vi "AlliGator Fit Decay.vi"(0 "Selected Plot Info + Flag":T13={"Multiplot XY Graph"=refnum, "Mouse Coordinates"={"Horizontal"=0, "Vertical"=0}, "Plot Index"=-1, "Flag"=FALSE}, 1 "Decay Fit Options & Parameters":T2 {"Fit Options"."Offset Resolution" min=0.0; "Fit Options"."Period" min=0.0; "Fit Options"."Min Decay Percentile" min=0.0 max=1.0; "Fit Options"."Max Decay Percentile" min=0.0 max=100.0; "Fit Parameter Constraints"."Max Value" format="%#.3g"; "Fit Parameter Constraints"."Min Value" format="%#.3g"}, 5 "Current Decay Name":string, 7 "Current Decay":T16, 9 "Reference Decay":T16, 11 "error in (no error)":errorcluster, 12 "Use Legacy Fitting Approach":bool) -> (2 "Decay Fit Options & Parameters (out)":T2 {"Fit Options"."Offset Resolution" min=0.0; "Fit Options"."Period" min=0.0; "Fit Options"."Min Decay Percentile" min=0.0 max=1.0; "Fit Options"."Max Decay Percentile" min=0.0 max=100.0; "Fit Parameter Constraints"."Max Value" format="%#.3g"; "Fit Parameter Constraints"."Min Value" format="%#.3g"}, 3 "Output Plots":T1(array[cluster]), 4 "Best Fit Parameters (All)":dbl[](array[numeric]), 6 "Delta Best Fit Parameters (All)":dbl[](array[numeric]), 8 "R^2":dbl, 10 "Reduced Chi^2":dbl, 13 "Output Plot Names":string[](array[string]), 14 "Fit Output Message":string, 15 "Error Out":errorcluster)   [LabVIEW 2021, in "AlliGator Decay Analysis.lvlib" / "AlliGator Decay Fit.lvlib"]
doc: "VI implementing single decay fit with either a single or double exponential model with IRF convolution (or in the absence of IRF, without convolution)."
uses:
  AlliGator Decay Fit.lvlib
  <vilib>/Analysis/Matrix/Datatypes/RealMatrix.ctl
  Graphs/XY Graph/XY Graph Selected Plot Info+Flag.ctl
  Graphs/XY Graph/XY Graph Refnum.ctl
  <vilib>/Utility/miscctls.llb/LVPoint32TypeDef.ctl
  AlliGator Decay Fit Options & Parameters v2.ctl
  Fits/IRF(X)PSED/Decay Fit Options v2.ctl
  Fits/Decay Convolution/Decay Model.ctl
  Fits/Residual Type.ctl
  Fits/IRF(X)PSED/Fit Weights Type.ctl
  Fits/Non-linear Fitting Method v2.ctl
  Fits/Fit Calculation Method.ctl
  Fits/Non-linear Fitting Algorithm.ctl
  AlliGator Decay Fit Parameter Constraints 2.ctl
  Fits/IRF(X)PSED/Decay Fit Parameters In List.ctl
  Fits/IRF(X)PSED/MLE Baseline Offset Type.ctl
  AlliGator Settings List.ctl
  AlliGator Variables List.ctl
  Fits/IRF(X)PSED/MLE Fit Options.ctl
  Graphs/Get Plot at Mouse Click (XY Graph)/Get Plot at Mouse Click [AAC].vi
  <vilib>/Utility/error.llb/Error Cluster From Error Code.vi
  Fits/Decay Convolution/LM model function and gradient (1-Exp, Convolved, Periodic, Fixed Parameters) v3.vi
  Fits/Decay Convolution/LM model function and gradient (2-Exp, Convolved, Periodic, Fixed Parameters) v3.vi
  Fits/Abort Fit Global.vi
  Graphs/XY Graph/XY Graph Add Multiplots with Names.vi
  <vilib>/ErrorRing/Error Ring.xnode
  Graphs/Graphs.lvlib
  Graphs/XY Graph/XY Graph Add-Ons.lvlib
  AlliGator Settings.lvlib
  Fits/Fits.lvlib
  AlliGator Globals, Variables & Constants.lvlib
  Time/Time.lvlib
  Strings/Strings.lvlib
  <vilib>/Analysis/Matrix/NI_Matrix.lvlib
  AlliGator Decay Fit Parameter Map.lvlib
panel:
  in  "Reset Fit Options & Parameters":bool
  out "Covariance":T17
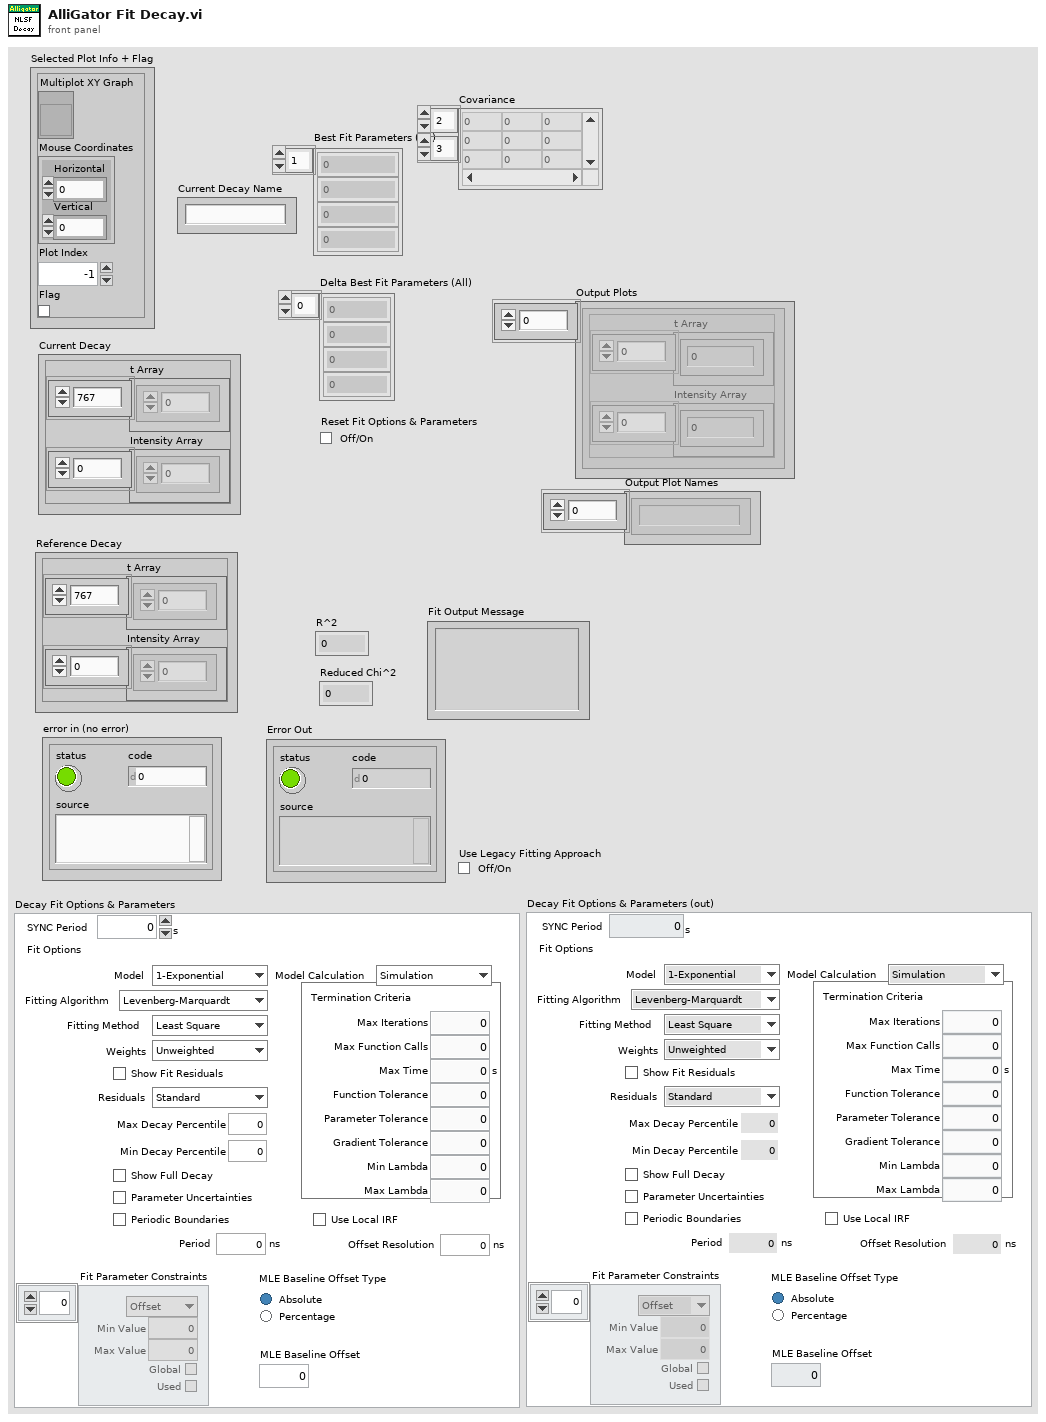
[diagram p1: front panel]
types:
  T1 = cluster{"t Array":dbl[], "Intensity Array":dbl[]}[]
  T2 = typedef "AlliGator Decay Fit Parameter Map.lvlib/AlliGator Decay Fit Options & Parameters v2.ctl" = cluster{"SYNC Period":dbl[unit], "Fit Options":T3, "Fit Parameter Constraints":T10[], "MLE Baseline Offset":dbl, "MLE Baseline Offset Type":T12}
  T3 = typedef "Fits.lvlib/Decay Fit Options v2.ctl" = cluster{"Show Fit Residuals":bool, "Fit Model":T4, "Residual Type":T5, "Max Decay Percentile":dbl, "Min Decay Percentile":dbl, "Show Full Decay":bool, "Weights":T6, "Fitting Method":T7, "Compute Parameter Uncertainties":bool, "Periodic Boundaries":bool, "Model Calculation":T8, "Period":dbl[unit], "Termination Criteria":cluster{"Max Iterations":i32, "Max Function Calls":i32, "Max Time":dbl[unit], "Function Tolerance":dbl, "Parameter Tolerance":dbl, "Gradient Tolerance":dbl, "Min Lambda":dbl, "Max Lambda":dbl, "Initial Tick Count":u32}, "Offset Resolution":dbl[unit], "Use Local IRF":bool, "Fitting Algorithm":T9}
  T4 = typedef "Fits.lvlib/Decay Model.ctl" = enum16{"1-Exponential", "2-Exponentials"}
  T5 = typedef "Fits.lvlib/Residual Type.ctl" = enum16{"Standard", "Normalized", "Reduced"}
  T6 = typedef "Fits.lvlib/Fit Weights Type.ctl" = enum16{"Unweighted", "1/Variance", "Best of All"}
  T7 = typedef "Fits.lvlib/Non-linear Fitting Method v2.ctl" = enum16{"Least Square", "Least Absolute Residual", "Bisquare", "MLE", "-", "Best of All"}
  T8 = typedef "Fits.lvlib/Fit Calculation Method.ctl" = enum16{"Simulation", "Convolution", "Integration"}
  T9 = typedef "Fits.lvlib/Non-linear Fitting Algorithm.ctl" = enum16{"Levenberg-Marquardt", "Trust-Region Dogleg"}
  T10 = typedef "AlliGator Decay Analysis.lvlib/AlliGator Decay Fit.lvlib/AlliGator Decay Fit Parameter Constraints 2.ctl" = cluster{"Fit Parameter":T11, "Min Value":dbl, "Max Value":dbl, "Global":bool, "Used":bool}
  T11 = typedef "Fits.lvlib/Decay Fit Parameters In List.ctl" = enum16{"Offset", "Baseline", "A_1", "tau_1", "A_2", "tau_2"}
  T12 = typedef "Fits.lvlib/MLE Baseline Offset Type.ctl" = enum32{"Absolute", "Percentage"}
  T13 = typedef "XY Graph Add-Ons.lvlib/XY Graph Selected Plot Info+Flag.ctl" = cluster{"Multiplot XY Graph":T14, "Mouse Coordinates":T15, "Plot Index":i32, "Flag":bool}
  T14 = typedef "XY Graph Add-Ons.lvlib/XY Graph Refnum.ctl" = refnum<vi>
  T15 = typedef "LVPoint32TypeDef.ctl" = cluster{"Horizontal":i32, "Vertical":i32}
  T16 = cluster{"t Array":dbl[], "Intensity Array":dbl[]}
  T17 = typedef "NI_Matrix.lvlib/RealMatrix.ctl" = dbl[][]
  T18 = typedef "AlliGator Settings.lvlib/AlliGator Settings List.ctl" = enum16{"GUI:Visible Settings Tab", "GUI:Last Run Version", "Source Image:Use Image Histogram for Contrast", "Source Image:Low Count Pixels Rejection Options", "Source Image:High Count Pixels Rejection Options", "Source Image:Use Image Brightness", "Source Image:Blend Overlay with Image Background", "Source Image:Use Fixed ROI Diameter", "Source Image:ROI Diameter", "Source Image:ROI Center Color", "Source Image:Peak Threshold", "Source Image:Intensity Threshold", "Source Image:Image Binning Options", "Source Image:Image Smoothing Options", "Source Image:Image Histogram Active", "Source Image:Invert Binary Mask", "Source Image:Hot Pixel Removal", "Source Image:Overlay Analyzed ROI Center", "Source Image:Auto-Adjust Contrast", "Source Image:Histogram Lower Percentile", "Source Image:Histogram Upper Percentile", "Source Image:Save Source Image", "Source Image:Scale Bar Options", "Source Image:Image Resolution (Pixel Size)", "Source Image:Flatfield Correction", "Source Image:Show Dead Left Columns Correction", "Source Image:Dead Left Columns Correction", "Source Image:Image Pre-Processing Operations Order", "Data Information:Gate Width", "Data Information:Nanotime Gate Separation", "Data Information:Macrotime Gate Separation", "Data Information:Gate Step", "Data Information:# Gates", "Data Information:Gate Image Exposure", "Data Information:Gate Image Integration", "Data Information:Gates to Skip", "Data Information:Gates to Keep", "Data Information:Define Gates to", "Data Information:Channel Name", "Data Information:Available Channel Names", "Data Information:Channel Arithmetic", "Data Information:Background File Subtraction", "Data Information:Background File", "Data Information:Background Scaling Factor", "Data Information:Background Pile-up Correction", "Data Information:Background Pixel Well Capacity", "Data Information:Laser Period", "Data Information:SYNC Period", "Data Information:Pile-up Correction", "Data Information:Pixel Well Capacity", "Data Information:Dataset Scaling Factor", "Fluorescence Decay_Decay Pre-Processing:Reverse Gates", "Fluorescence Decay_Decay Pre-Processing:Verbose Decay Pre-Processing", "Fluorescence Decay_Decay Pre-Processing:Use Decay Pre-Processing", "Fluorescence Decay_Decay Pre-Processing:Background Subtraction", "Fluorescence Decay_Decay Pre-Processing:Background Definition Range", "Fluorescence Decay_Decay Pre-Processing:Baseline Subtraction Method", "Fluorescence Decay_Decay Pre-Processing:Decay Pre-Processing Operations Order", "Fluorescence Decay_Decay Pre-Processing:Smoothing Parameter", "Fluorescence Decay_Decay Pre-Processing:Shift Decay", "Fluorescence Decay_Decay Pre-Processing:Decay Shift Parameters", "Fluorescence Decay_Decay Pre-Processing:Fold Decay", "Fluorescence Decay_Decay Pre-Processing:# Folds", "Fluorescence Decay_Decay Pre-Processing:1-Normalize Decay", "Fluorescence Decay_Decay Pre-Processing:[0-1]-Normalize Decay", "Fluorescence Decay_Decay Pre-Processing:Smoothen Decay", "Fluorescence Decay_Decay Pre-Processing:Extrapolate Decay", "Fluorescence Decay_Decay Pre-Processing:Use Periodicity", "Fluorescence Decay_Decay Pre-Processing:Use Cursors", "Fluorescence Decay_Decay Pre-Processing:Tail Fraction", "Fluorescence Decay_Decay Pre-Processing:Head Fraction", "Fluorescence Decay_Decay Pre-Processing:Additional Points", "Fluorescence Decay_Decay Pre-Processing:Straighten Decay", "Fluorescence Decay_Decay Pre-Processing:Constant Background", "Fluorescence Decay_Decay Pre-Processing:Pixel-Normalize Decay", "Fluorescence Decay_Advanced Analysis:Extract IRF instead of Decay", "Fluorescence Decay_Advanced Analysis:IRF Extraction Options", "Fluorescence Decay_Advanced Analysis:IRF Optimization Options", "Fluorescence Decay_Advanced Analysis:Square Pulse Options", "Fluorescence Decay_Advanced Analysis:IRF Order", "Fluorescence Decay_Advanced Analysis:IRF Time Constants", "Fluorescence Decay_Advanced Analysis:Wavelet Analysis Options", "Fluorescence Decay_Advanced Analysis:Average Lifetime Options", "Fluorescence Decay_Fit Options:Fit Options", "Fluorescence Decay_Fit Options:Use Legacy Fitting Approach", "Fluorescence Decay_Fit Options:Use Data Information Laser Period", "Fluorescence Decay_Fit Parameters:Displayed Fit Parameters", "Fluorescence Decay_Fit Parameters:Fit Parameter Constraints", "Fluorescence Decay_Fit Parameters:Export Tabulated Results", "Fluorescence Decay_Fit Parameters:MLE Baseline Offset Type", "Fluorescence Decay_Fit Parameters:MLE Baseline Offset", "Fluorescence Decay_Fit Parameters:Guess Parameter Names", "Fluorescence Decay_Fit Parameters:Guess Parameter Values", "Fluorescence Decay_Fit Parameters:Guess Parameters Options", "Fluorescence Decay_Styles:Show Last Decay Only", "Fluorescence Decay_Styles:Decay Graph Color Array", "Fluorescence Decay:Decay Graph Active", "Fluorescence Decay Statistics:Min Peak Value", "Fluorescence Decay Statistics:Reject Low Decay Peak Pixels", "Fluorescence Decay Statistics:Reject High Decay Peak Pixels", "Fluorescence Decay Statistics:Max Peak Value", "Time Traces:Use File Timestamp", "Time Traces:Time Step", "Time Traces:Use Intensity Correction File", "Time Traces:Intensity Correction File", "Phasor Plot:Phasor Plot Smoothing Options", "Phasor Plot:Phasor Plot Size", "Phasor Plot:Phasor Plot Graphics Options", "Phasor Plot:Cumulative Phasor Plot", "Phasor Plot:Use Phasor Brightness", "Phasor Plot:Blend Overlay with Phasor Background", "Phasor Plot:Save Phasor Plot", "Phasor Plot:Show References", "Phasor Plot:Phasor Ratio Decay Range", "Phasor Plot:Exponential Fading", "Phasor Plot:Phasor Ratio Reference Colors", "Phasor Plot:Reference Radius", "Phasor Plot:Show Color Map Vertices", "Phasor Plot:Phasor Plot Active", "Phasor Plot:Phasor Ratio Color Map Type", "Phasor Plot:Phasor Ratio Color Map", "Phasor Plot:Phasor Ratio Display Range", "Phasor Plot:Selected Image ROI(s)", "Phasor Plot:All Image ROIs", "Phasor Plot:Selected Phasor Plot ROI(s)", "Phasor Plot:All Phasor Plot ROIs", "Phasor Plot:Phasor Ratio Color-Coded Quantity", "Phasor Plot:Store Phasor Harmonics", "Phasor Plot:Draw Reference Segment", "Phasor Plot:User-Defined Quantity", "Phasor Graph:Phasor Frequency", "Phasor Graph:Phasor Ratio Type", "Phasor Graph:Pixel-level Phasor Computation", "Phasor Graph:Save Phasor Graph", "Phasor Graph:Phasor Graph Active", "Phasor Graph:Phasor SDV Options", "Phasor Calibration:Use Backup Calibration if needed", "Phasor Graph:Define Shortest Lifetime as", "Phasor Calibration:Backup Calibration Type", "Phasor Calibration:Calibration Type", "Phasor Calibration:Calibration Lifetime", "Phasor Calibration:Calibration Map Algorithm", "Single-Exponential Phasor Locus (SEPL):Gate Parameters", "Single-Exponential Phasor Locus (SEPL):User-defined Gate", "Single-Exponential Phasor Locus (SEPL):User-defined IRF", "Single-Exponential Phasor Locus (SEPL):Phasor Parameters", "Single-Exponential Phasor Locus (SEPL):Decay & IRF Parameters", "Single-Exponential Phasor Locus (SEPL):Display Parameters", "Lifetime Analysis:Decay Analysis Parameters", "Lifetime Analysis:Lifetime Map Active", "Plugins:Python Settings", "Miscellaneous:Verbose Mode", "Miscellaneous:Beep after Script", "Miscellaneous:Saved Image File Format", "Miscellaneous:Exported Gate Image Settings", "Miscellaneous:Include Loading in Timing", "Miscellaneous:Verbose Settings Mode", "Miscellaneous:Histogram Options", "Miscellaneous:Beep on Error", "Miscellaneous:# Logical Processors Used", "Miscellaneous:ROI Description Max Characters", "Miscellaneous:Verbose Error Mode", "Miscellaneous:Transparent Mask Color"}
  T19 = cluster{"X Array out":dbl[], "Y Array out":dbl[]}
  T20 = typedef "AlliGator Globals, Variables & Constants.lvlib/AlliGator Variables List.ctl" = enum16{"---- GUI ----", "Initialization Status", "State Indicators Refnum", "Original AlliGator Menu Items", "Current Action Loop State", "Script in progress", "Playback", "Loop Playback", "Search ROI Used", "Search ROI", "Decay Graph Max Legend Size", "Intensity Graph Max Legend Size", "Decay Statistics Graph Max Legend Size", "Phasor Graph Max Legend Size", "Phasor Ratio Graph Max Legend Size", "Lifetime Graph Max Legend Size", "---- Files ----", "Export Dataset Frames as Individual Files", "Show Batch Export Help Balloons", "Frames in Dataset", "ptu File Frame Start Indices", "Current Frame in Dataset", "Current Frame Timestamp", "------ Python Plugins ------", "Python Plugins Information", "Python Session", "Valid Python Session?", "---- Source Image ----", "Dataset Loaded", "Dataset Metadata", "Dataset Channel", "Dataset Data Description", "Background Dataset Metadata", "Background Dataset Channel", "Background Dataset Data Description", "Background File Subtraction", "Background File Path", "Background File Pile-up Correction", "Background File Pixel Well Capacity", "Background File Scaling Factor", "Source Image ROIs", "Current Source Image ROI", "Source Image ROI Event Refnum", "X_Source Image Display Range", "X_Source Image Palette Information", "Source Image Palette List", "Source Image Scale", "Current Dataset Load Settings", "Source Image:ROI Overlay Color", "---- Image Profile Window ----", "Image Profile:Overlay ROI in Source Image", "Image Profile Window Event Refnum", "Image Profile:IntensityType", "Image Profile:Intensity Average Type", "Image Profile:Intensity-weighted SDV", "Image Profile:Box Profile Type", "Image Profile Window Open", "Image Profile:Plotted Fit Parameter", "X_Type of Displayed Image", "X_Time Gate Slider", "Dataset Path", "Source Image Overlay to Erase", "Is Displayed Image Accumulated", "White Light Image Modified", "Mask Image Modified", "Macrotime Gate Separation", "------ Phasor Graph -------", "Phasor Graph:Show Line", "---- Phasor Plot ---", "Phasor Plot Parameters Changed", "FLI Dataset Modified since last Phasor Plot Calculation", "Phasor Harmonics Data", "Selected Phasor Harmonics", "Phasor Harmonic Manager Event Refnum", "Phasor Plot ROIs", "Current Phasor Plot ROI", "Phasor Plot ROI Event Refnum", "Phasor Plot Image Reference Points", "Phasor Plot Computed", "Phasor Plot Palette Information", "Phasor Plot Palette List", "Phasor Ratio Palette Information", "Phasor Ratio Palette List", "Phasor Image Scale", "Phasor Plot Image Overlay to Erase", "Phasor Plot Image Elements to Update", "Current Phasor Plot Calculation Parameters", "Current Phasor Calibration Options", "Reset Cumulated Phasor Plot", "Phasor Ratio Reference 1", "Phasor Ratio Lifetime Reference 1", "Phasor Ratio Reference 1 Frequency", "Phasor Ratio Reference 2", "Phasor Ratio Lifetime Reference 2", "Phasor Ratio Reference 2 Frequency", "---- Decay Analysis ----", "Number of Selected Decays to Fit", "LS Fit Results", "LAR Fit Results", "BS Fit Results", "Last Decay Max - Min", "Best Fit Parameters", "Best Fit Parameter Names", "Actual Size X", "Actual Size Y", "Binning X", "Binning Y", "Actual # Gates", "Dataset Number", "Gates to...", "Gates Skipped", "Gates to keep", "Gate Step", "Gate Separation", "Reversed Gates", "Pile-up Correction", "Pixel Well Capacity", "Background Subtracted", "Background Subtraction Method", "Background Definition Range", "Background File (deprecated)", "Number of Dataset Accumulated", "Array of Accumulated Dataset Paths", "Do Averaged Datasets", "Destination File Path", "Process Plot Target", "Use 1/D as Phasor Frequency", "---- Decay Fit Parameter Map -----", "Decay Fit Parameter Map Palette Information", "Decay Fit Parameter Map Palette List", "Local Decay Graph Window Event Refnum", "------- Local Decay Window ---------", "Use normalized IRF for convolution", "----- Miscellaneous ----", "Skippable Dialog Windows Status"}
  T21 = typedef "Fits.lvlib/MLE Fit Options.ctl" = cluster{"MLE Baseline Offset":dbl, "MLE Baseline Offset Type":T12}
  T22 = typedef "Fits.lvlib/Decay Fit Parameter Constraints Arrays.ctl" = cluster{"Parameter Bounds (Fix+Fit)":cluster{"parameter minimum":dbl[], "parameter maximum":dbl[]}, "Fitted Parameters":T11[], "Fixed Parameters":T11[], "Fit Model":T4}
  T23 = typedef "Graphs.lvlib/Plot Range.ctl" = cluster{"X Minimum":dbl, "X Maximum":dbl, "Y Minimum":dbl, "Y Maximum":dbl}
  T24 = cluster{"parameter minimum":dbl[], "parameter maximum":dbl[]}
  T25 = typedef "Fits.lvlib/Non-linear Fit Output v3.ctl" = cluster{"best nonlinear fit":dbl[], "best fit parameters":dbl[], "R^2":dbl, "RMSE":dbl, "error out":errorcluster, "Fitting Method":T26, "number of function calls":i32, "number of iterations":i32, "covariance":T17, "Chi 2":dbl, "DOF":i32, "Fit Convergence Criterion":T27, "Fitting Algorithm":T9, "Weighted Fit":bool, "Gradient":dbl, "|Delta Chi 2|":dbl, "|Delta Chi 2|/Chi 2":dbl, "Max |Delta a| /|a|":dbl, "Lambda":dbl, "RSS":dbl, "AIC":dbl, "BIC":dbl, "Max number of function calls":i32, "Max number of iterations":i32, "IRF":T28, "IRF Normalization Factor":dbl, "Decay Normalization Factor":dbl}
  T26 = typedef "Fits.lvlib/Nonlinear Fit Method.ctl" = enum16{"Least Square", "Least Absolute Residual", "Bisquare", "MLE"}
  T27 = typedef "Fits.lvlib/Convergence Criteria.ctl" = enum16{"Continue", "Tolerances Exceeded", "Max Time Exceeded", "Max Iterations Exceeded", "Max Function Evaluations Exceeded", "Scale Range Exceeded"}
  T28 = typedef "XY Graph Add-Ons.lvlib/XY Plot Data.ctl" = cluster{"X Array":dbl[], "Y Array":dbl[]}
  T29 = typedef "AlliGator Decay Analysis.lvlib/AlliGator Decay Fit.lvlib/AlliGator Guess Parameters Options.ctl" = enum16{"Numerically estimated", "User-provided", "User-provided (normalized)", "Last valid fitted parameters"}
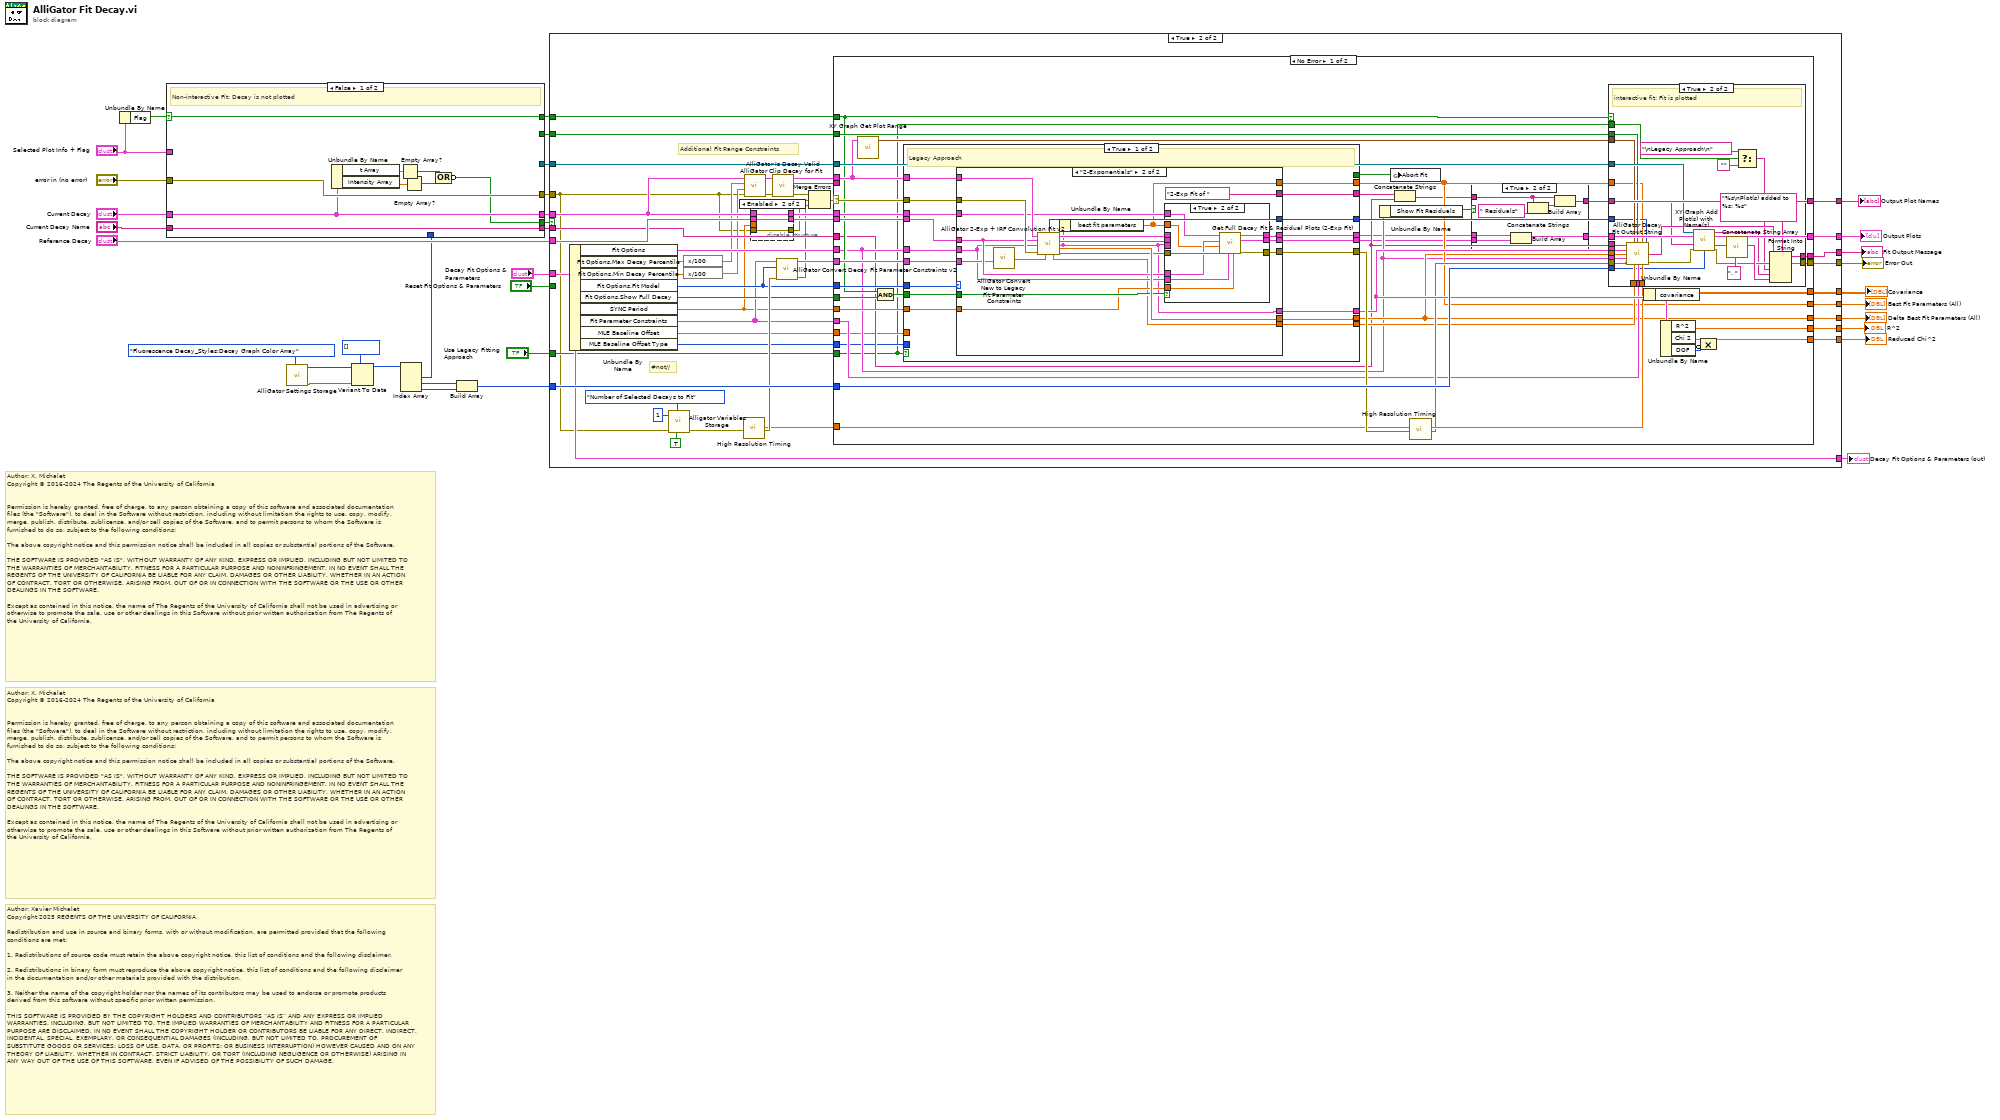
[diagram p0: block diagram]
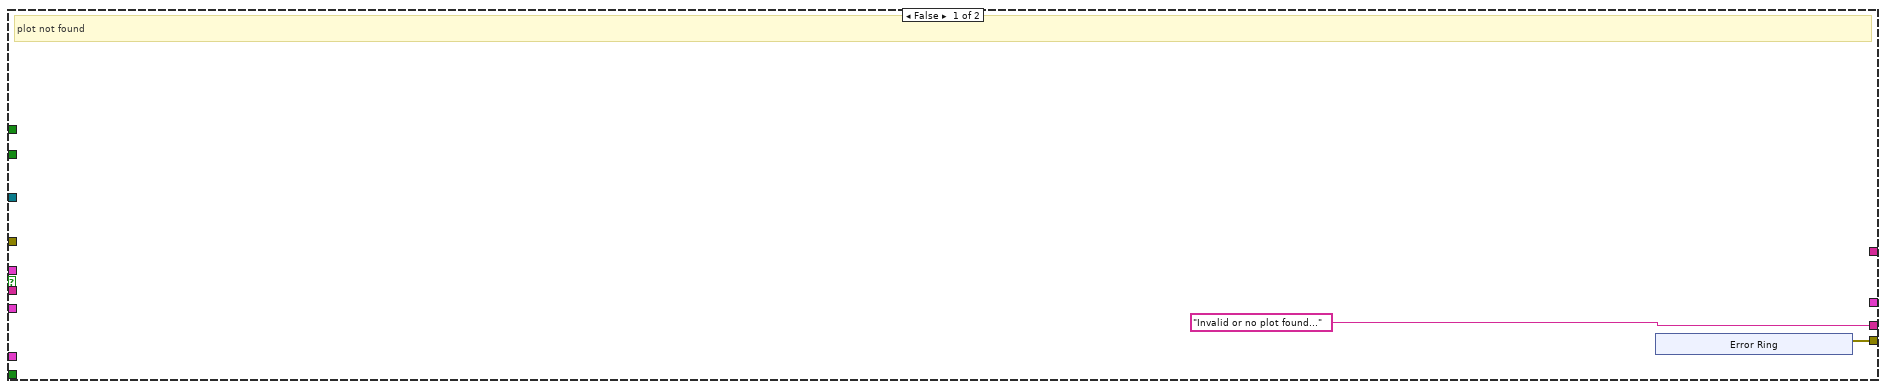
[diagram p2: hidden frame]
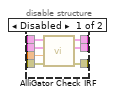
[diagram p3: hidden frame]
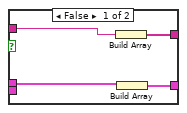
[diagram p5: hidden frame]
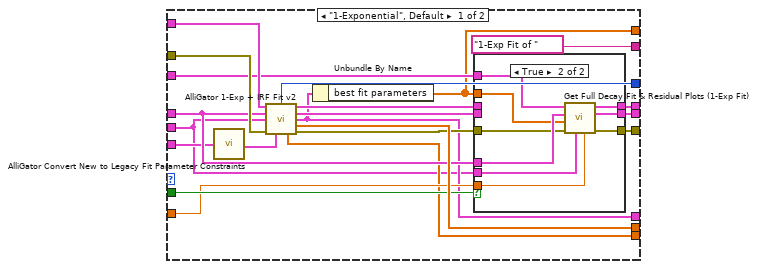
[diagram p6: hidden frame]
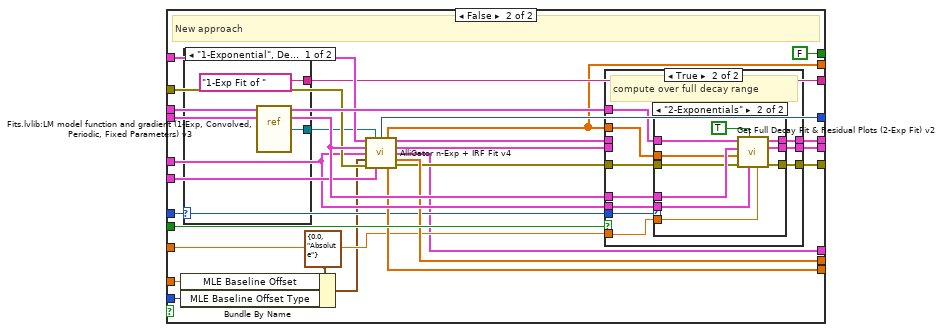
[diagram p9: hidden frame]
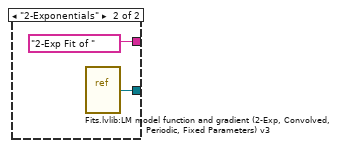
[diagram p10: hidden frame]
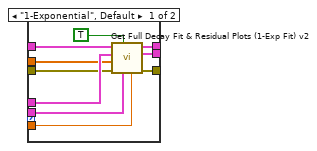
[diagram p12: hidden frame]
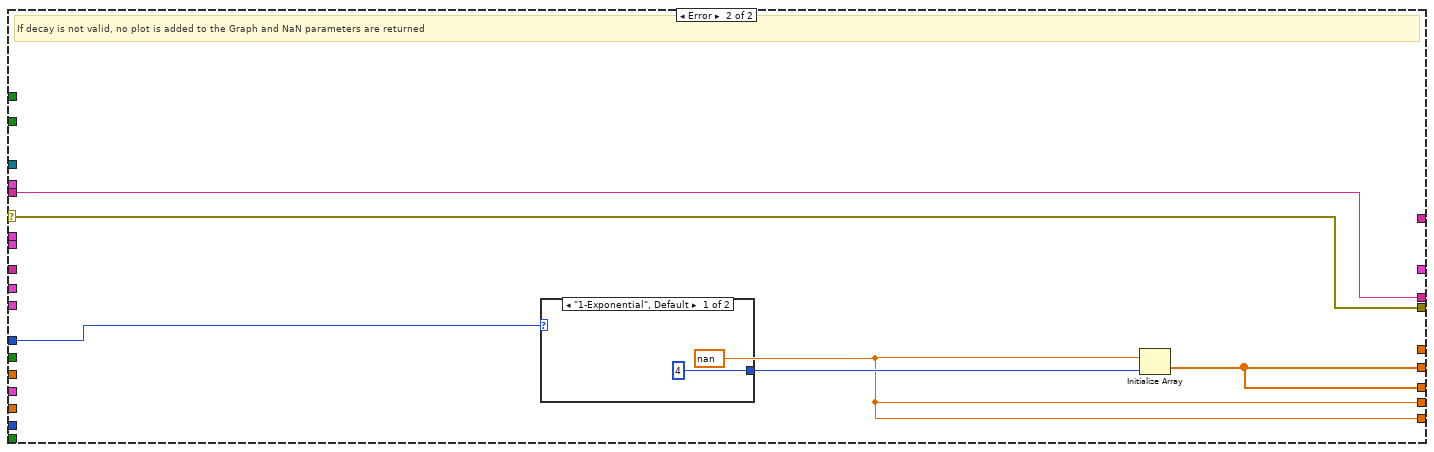
[diagram p13: hidden frame]
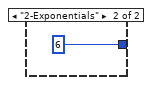
[diagram p14: hidden frame]
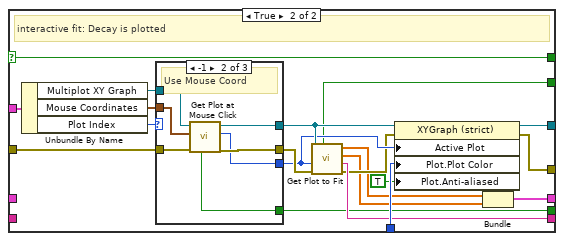
[diagram p15: hidden frame]
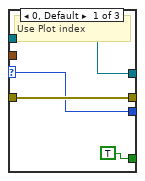
[diagram p16: hidden frame]
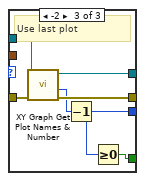
[diagram p17: hidden frame]
diagram:
  # "Author: Xavier Michalet\nCopyright 2025 REGENTS OF THE UNIVERSITY OF CALIFORNIA\n\nRedistribution and use in source and binary forms, with or without modification, are permitted provided that the following conditions are met:\n\n1. Redistributions of source code must retain the above copyright notice, this list of conditions and the following disclaimer.\n\n2. Redistributions in binary form must reproduce the above copyright notice, this list of conditions and the following disclaimer in the documentation and/or other materials provided with the distribution.\n\n3. Neither the name of the copyright holder nor the names of its contributors may be used to endorse or promote products derived from this software without specific prior written permission.\n\nTHIS SOFTWARE IS PROVIDED BY THE COPYRIGHT HOLDERS AND CONTRIBUTORS “AS IS” AND ANY EXPRESS OR IMPLIED WARRANTIES, INCLUDING, BUT NOT LIMITED TO, THE IMPLIED WARRANTIES OF MERCHANTABILITY AND FITNESS FOR A PARTICULAR PURPOSE ARE DISCLAIMED. IN NO EVENT SHALL THE COPYRIGHT HOLDER OR CONTRIBUTORS BE LIABLE FOR ANY DIRECT, INDIRECT, INCIDENTAL, SPECIAL, EXEMPLARY, OR CONSEQUENTIAL DAMAGES (INCLUDING, BUT NOT LIMITED TO, PROCUREMENT OF SUBSTITUTE GOODS OR SERVICES; LOSS OF USE, DATA, OR PROFITS; OR BUSINESS INTERRUPTION) HOWEVER CAUSED AND ON ANY THEORY OF LIABILITY, WHETHER IN CONTRACT, STRICT LIABILITY, OR TORT (INCLUDING NEGLIGENCE OR OTHERWISE) ARISING IN ANY WAY OUT OF THE USE OF THIS SOFTWARE, EVEN IF ADVISED OF THE POSSIBILITY OF SUCH DAMAGE."
  # "Author: X. Michalet\nCopyright © 2016-2024 The Regents of the University of California\n \n\nPermission is hereby granted, free of charge, to any person obtaining a copy of this software and associated documentation files (the \"Software\"), to deal in the Software without restriction, including without limitation the rights to use, copy, modify, merge, publish, distribute, sublicense, and/or sell copies of the Software, and to permit persons to whom the Software is furnished to do so, subject to the following conditions:\n\nThe above copyright notice and this permission notice shall be included in all copies or substantial portions of the Software.\n\nTHE SOFTWARE IS PROVIDED \"AS IS\", WITHOUT WARRANTY OF ANY KIND, EXPRESS OR IMPLIED, INCLUDING BUT NOT LIMITED TO THE WARRANTIES OF MERCHANTABILITY, FITNESS FOR A PARTICULAR PURPOSE AND NONINFRINGEMENT. IN NO EVENT SHALL THE REGENTS OF THE UNIVERSITY OF CALIFORNIA BE LIABLE FOR ANY CLAIM, DAMAGES OR OTHER LIABILITY, WHETHER IN AN ACTION OF CONTRACT, TORT OR OTHERWISE, ARISING FROM, OUT OF OR IN CONNECTION WITH THE SOFTWARE OR THE USE OR OTHER DEALINGS IN THE SOFTWARE.\n\nExcept as contained in this notice, the name of The Regents of the University of California shall not be used in advertising or otherwise to promote the sale, use or other dealings in this Software without prior written authorization from The Regents of the University of California."
  # "Author: X. Michalet\nCopyright © 2016-2024 The Regents of the University of California\n \n\nPermission is hereby granted, free of charge, to any person obtaining a copy of this software and associated documentation files (the \"Software\"), to deal in the Software without restriction, including without limitation the rights to use, copy, modify, merge, publish, distribute, sublicense, and/or sell copies of the Software, and to permit persons to whom the Software is furnished to do so, subject to the following conditions:\n\nThe above copyright notice and this permission notice shall be included in all copies or substantial portions of the Software.\n\nTHE SOFTWARE IS PROVIDED \"AS IS\", WITHOUT WARRANTY OF ANY KIND, EXPRESS OR IMPLIED, INCLUDING BUT NOT LIMITED TO THE WARRANTIES OF MERCHANTABILITY, FITNESS FOR A PARTICULAR PURPOSE AND NONINFRINGEMENT. IN NO EVENT SHALL THE REGENTS OF THE UNIVERSITY OF CALIFORNIA BE LIABLE FOR ANY CLAIM, DAMAGES OR OTHER LIABILITY, WHETHER IN AN ACTION OF CONTRACT, TORT OR OTHERWISE, ARISING FROM, OUT OF OR IN CONNECTION WITH THE SOFTWARE OR THE USE OR OTHER DEALINGS IN THE SOFTWARE.\n\nExcept as contained in this notice, the name of The Regents of the University of California shall not be used in advertising or otherwise to promote the sale, use or other dealings in this Software without prior written authorization from The Regents of the University of California."
  n1 = Unbundle By Name("Selected Plot Info + Flag") -> ("Flag"=w12:bool)
  n2 = call "AlliGator Settings Storage.vi"("AlliGator Settings List"=AlliGator_Settings_List."Fluorescence Decay_Styles:Decay Graph Color Array") -> ("Error Out"=w26:errorcluster, "Variant Data out"=w27:variant)  [unwired: 9 in]
  n3 = Variant To Data(error in=w26, type=u32[] [] ("appended array"), Variant=w27) -> (data=w24:u32[])  [unwired: 1 out]
  n4 = Index Array(array=w24) -> (element #1=w23:u32, element #2=w7:u32, element #3=w6:u32)  [unwired: 3 in]
  n5 = case shown="False" w12 {
    selector: w12 -> [w36 w45]
    tunnel: w23 -> [_ w61]
    tunnel: "error in (no error)" -> [w44 w60]
    tunnel: [_ w59] -> w21
    tunnel: [w44 w58] -> w20
    tunnel: [w42 w57] -> w19
    tunnel: [w43 w56] -> w18
    tunnel: [_ w55] -> w17
    tunnel: "Current Decay" -> [w42 _]
    tunnel: "Current Decay Name" -> [w43 _]
    tunnel: [w37 w51] -> w14
    tunnel: "Selected Plot Info + Flag" -> [_ w50]
    tunnel: [w36 w45] -> w11
    frame False {
      # "Non-interactive Fit: Decay is not plotted"
      n6 = Unbundle By Name(w42) -> ("t Array"=w41:dbl[], "Intensity Array"=w40:dbl[])
      n7 = Empty Array?(array=w41) -> (empty?=w39:bool)
      n8 = Empty Array?(array=w40) -> (empty?=w38:bool)
      n9 = Compound Arithmetic op=OR(w39, w38) -> (invert w37:bool)
    }
    frame True {
      # "interactive fit: Decay is plotted"
      n10 = Unbundle By Name(w50) -> ("Multiplot XY Graph"=w49:T14, "Mouse Coordinates"=w47:T15, "Plot Index"=w48:i32)
      n11 = case shown="-1" w48 {
        selector: w48 -> [w65 _ _]
        tunnel: w60 -> [w68 w75 w81]
        tunnel: [w66 w74 w82] -> w64
        tunnel: [w68 w73 w80] -> w63
        tunnel: [w65 w72 w78] -> w62
        tunnel: [TRUE ("Found?") w71 w77] -> w51
        tunnel: w49 -> [w66 w70 w76]
        tunnel: w47 -> [_ w69 _]
        frame 0, Default {
          # "Use Plot index"
        }
        frame -1 {
          # "Use Mouse Coord"
          n12 = call-poly "Get Plot at Mouse Click.vi"("error in (no error)"=w75, "Mouse Click Coordinates"=w69, "XYGraph Ref"=w70) -> ("error out"=w73:errorcluster, "Plot at Coordinates"=w72:i32, "XYGraph Ref"=w74:T14, "Found?"=w71:bool)  [unwired: 2 in, 3 out]
        }
        frame -2 {
          # "Use last plot"
          n13 = call "XY Graph Get Plot Names & Number.vi"("error in (no error)"=w81, "XYGraph in"=w76) -> ("error out"=w80:errorcluster, "# Plots"=w79:i32, "XYGraph out"=w82:T14)  [unwired: 4 in, 3 out]
          n14 = Decrement(x=w79) -> (x-1=w78:i32)
          n15 = Greater Or Equal To 0?(x=w78) -> (x >= 0?=w77:bool)
        }
      }
      n16 = call "Get Plot to Fit.vi"("error in (no error)"=w63, "Plot Index"=w62, "XYGraph in"=w64) -> ("error out"=w54:errorcluster, "Plot Name"=w56:string, "Y Array out"=w52:dbl[], "X Array out"=w53:dbl[], "Plot clipped?"=w55:bool)  [unwired: 2 in, 2 out]
      n17 = property class="XYGraph (strict)"(reference=w64, error in=w54, "Active Plot"=w62, "Plot.Plot Color"=w61, "Plot.Anti-aliased"=TRUE) -> (reference out=w59:T14, error out=w58:errorcluster)
      n18 = Bundle("X Array out"=w53, "Y Array out"=w52) -> (w57:T19)  [unwired: 1 in]
    }
  }
  n19 = Build Array(w7, w6) -> (w5:u32[])
  n20 = case shown="True" w14 {
    tunnel: [w84 w135] -> w35
    tunnel: ["Invalid or no plot found..." ("Message") w114] -> w34
    tunnel: [_ w134] -> w33
    tunnel: [_ w133] -> w32
    tunnel: [_ w132] -> w31
    tunnel: [_ w131] -> w30
    tunnel: "Reference Decay" -> [_ w130]
    tunnel: w5 -> [_ w129]
    tunnel: [_ w128] -> w22
    tunnel: w21 -> [_ w127]
    tunnel: w20 -> [_ w92]
    tunnel: w19 -> [_ w126]
    tunnel: w18 -> [_ w120]
    tunnel: w17 -> [_ w117]
    tunnel: w11 -> [_ w116]
    tunnel: "Reset Fit Options & Parameters" -> [_ _]
    tunnel: [_ w104] -> w8
    tunnel: "Decay Fit Options & Parameters" -> [_ w104]
    tunnel: "Use Legacy Fitting Approach" -> [_ w103]
    tunnel: [_ w96] -> w1
    tunnel: [_ w95] -> w2
    frame False {
      # "plot not found"
      n21 = xnode "Error Ring"() -> ("error out"=w84:errorcluster)
    }
    frame True {
      # "#not//"
      # "Additional Fit Range Constraints"
      n22 = Unbundle By Name(w104) -> ("Fit Options"=w106:T3, "Fit Options.Max Decay Percentile"=w109:dbl, "Fit Options.Min Decay Percentile"=w101:dbl, "Fit Options.Fit Model"=w108:T4, "Fit Options.Show Full Decay"=w107:bool, "SYNC Period"=w97:dbl[unit], "Fit Parameter Constraints"=w105:T10[], "MLE Baseline Offset"=w94:dbl, "MLE Baseline Offset Type"=w93:T12)
      n23 = call "Alligator Variables Storage.vi"("Get(F)/Set"=TRUE, "AlliGator Variable"=AlliGator_Variables_List."Number of Selected Decays to Fit" ("Alligator Variable"), "Error In"=w92, "Data in"=1) -> ("Error Out"=w110:errorcluster)  [unwired: 5 in, 2 out]
      n24 = expression code="x/100"(w109) -> (w102:dbl)
      n25 = expression code="x/100"(w101) -> (w100:dbl)
      n26 = call "High Resolution Timing.vi"("Error In"=w110) -> ("elapsed (relative) seconds"=w118:dbl, "Error Out"=w119:errorcluster)  [unwired: 16 in, 1 out]
      n27 = call "AlliGator Clip Decay for Fit.vi"("Error In"=w92, "Min Decay Percentile (0)"=w100, "Max Decay Percentile (1)"=w102, "Decay in"=w126) -> ("Error Out"=w124:errorcluster, "Clipped Decay out"=w115:cluster{"t Array":dbl[], "Value Array":dbl[]})  [unwired: 3 in, 3 out]
      n28 = disable-structure shown="Enabled" {
        disable-tunnel: w130 -> [w142 w144]
        disable-tunnel: w126 -> [w141 w145]
        disable-tunnel: [w140 w145] -> w99
        disable-tunnel: [w139 w144] -> w98
        disable-tunnel: w97 -> [w138 _]
        disable-tunnel: w92 -> [w137 w143]
        disable-tunnel: [w136 w143] -> w90
        frame Disabled {
          n29 = call "AlliGator Check IRF.vi"("Error In"=w137, "SYNC Period"=w138, "Reference Decay"=w142, "Current Decay"=w141) -> ("Error Out"=w136:errorcluster, "Reference Decay (or Dirac)"=w139:cluster{"t Array":dbl[], "IRF Array":dbl[]}, "Current Decay (dup)"=w140:T16)  [unwired: 5 in]
        }
        frame Enabled {
        }
      }
      n30 = call "AlliGator Is Decay Valid.vi"("Error In"=w124, "Decay"=w115) -> ("Error Out"=w123:errorcluster, "Message"=w122:string, "Decay (dup)"=w125:cluster{"t Array":dbl[], "Value Array":dbl[]})  [unwired: 6 in, 1 out]
      n31 = call "AlliGator Convert Decay Fit Parameter Constraints v2.vi"("Error In"=w119, "Fit Model"=w108, "Fit Parameter Constraints"=w105) -> ("Error Out"=w89:errorcluster, "All Parameter Constraints"=w121:T22)  [unwired: 6 in, 1 out]
      n32 = Merge Errors(w123, w90, w89) -> (w91:errorcluster)
      n33 = case shown="No Error" w91 {
        selector: w91 -> [w184 w385]
        tunnel: w127 -> [w189 _]
        tunnel: [w188 w385] -> w135
        tunnel: [w160 w382] -> w134
        tunnel: [w159 w382] -> w133
        tunnel: [w179 w381] -> w132
        tunnel: w108 -> [w182 w384]
        tunnel: [w163 w381] -> w131
        tunnel: w98 -> [w187 _]
        tunnel: w107 -> [w186 _]
        tunnel: w99 -> [w185 _]
        tunnel: w125 -> [w174 _]
        tunnel: w120 -> [w156 _]
        tunnel: w106 -> [w158 _]
        tunnel: w122 -> [_ w380]
        tunnel: w129 -> [w183 _]
        tunnel: w121 -> [w181 _]
        tunnel: w105 -> [w164 _]
        tunnel: [w177 _] -> w128
        tunnel: w118 -> [w175 _]
        tunnel: w97 -> [w176 _]
        tunnel: w117 -> [w172 _]
        tunnel: w116 -> [w166 _]
        tunnel: [w169 w380] -> w114
        tunnel: w103 -> [w146 _]
        tunnel: [w150 _] -> w96
        tunnel: [w149 _] -> w95
        tunnel: w94 -> [w148 _]
        tunnel: w93 -> [w147 _]
        frame No Error {
          n34 = call "XY Graph Get Plot Range.vi"("Plot in"=w174) -> ("Plot Range"=w173:T23)  [unwired: 10 in]
          n35 = Compound Arithmetic op=AND(w166, w186) -> (w167:bool)
          n36 = case shown="True" w146 {
            tunnel: [w249 w342] -> w152
            tunnel: w187 -> [w248 w341]
            tunnel: w185 -> [w247 w340]
            tunnel: w184 -> [w246 w339]
            tunnel: w182 -> [w245 w324]
            tunnel: w181 -> [w244 w338]
            tunnel: [w243 w337] -> w180
            tunnel: [w242 w336] -> w151
            tunnel: w176 -> [w241 w322]
            tunnel: w174 -> [w240 w335]
            tunnel: [w239 w317] -> w171
            tunnel: w158 -> [w238 w334]
            tunnel: [w237 w333] -> w157
            tunnel: w167 -> [w236 w332]
            tunnel: [w235 w331] -> w165
            tunnel: [w234 w330] -> w161
            tunnel: [w233 w316] -> w160
            tunnel: [w232 w329] -> w159
            tunnel: [_ FALSE ("Abort Fit")] -> w155
            tunnel: w148 -> [_ w321]
            tunnel: w147 -> [_ w320]
            frame True {
              # "Legacy Approach"
              n37 = case shown="\"2-Exponentials\"" w245 {
                tunnel: w248 -> [w260 w292]
                tunnel: w246 -> [w270 w303]
                tunnel: ["1-Exp Fit of " ("string") "2-Exp Fit of " ("string")] -> w237
                tunnel: w240 -> [w264 w294]
                tunnel: [w265 w297] -> w249
                tunnel: [w262 w295] -> w243
                tunnel: [w268 w301] -> w232
                tunnel: w236 -> [w267 w300]
                tunnel: w247 -> [w261 w293]
                tunnel: w238 -> [w250 w288]
                tunnel: w244 -> [w259 w291]
                tunnel: [w257 w290] -> w242
                tunnel: [w255 w287] -> w239
                tunnel: w241 -> [w256 w289]
                tunnel: [w253 w284] -> w234
                tunnel: [w254 w286] -> w235
                tunnel: [w252 w285] -> w233
                frame "1-Exponential", Default {
                  n38 = call "AlliGator Convert New to Legacy Fit Parameter Constraints.vi"("All Parameter Constraints"=w259) -> ("Parameter Bounds"=w251:T24)
                  n39 = call "AlliGator 1-Exp + IRF Fit v2.vi"("Decay"=w264, "IRF"=w260, "Fit Options"=w250, "error in (no error)"=w270, "parameter bounds"=w251) -> ("Fitted Decay"=w266:cluster{"t Array":dbl[], "Fitted Array":dbl[]}, "Residuals"=w258:cluster{"t Array":dbl[], "Residual Array":dbl[]}, "Fit Output"=w255:T25, "Delta Best Fit Parameters"=w268:dbl[], "Guess Parameters Options"=w254:T29, "Guess Parameters"=w253:dbl[], "error out"=w263:errorcluster)  [unwired: 4 in]
                  n40 = Unbundle By Name(w255) -> ("best fit parameters"=w252:dbl[])
                  n41 = case shown="True" w267 {
                    tunnel: w266 -> [w273 _]
                    tunnel: [w273 w278] -> w265
                    tunnel: w260 -> [_ w282]
                    tunnel: w261 -> [_ w281]
                    tunnel: w263 -> [w272 w280]
                    tunnel: [w272 w279] -> w262
                    tunnel: [w271 w277] -> w257
                    tunnel: w258 -> [w271 _]
                    tunnel: w256 -> [_ w275]
                    tunnel: w250 -> [_ w276]
                    tunnel: w252 -> [_ w274]
                    frame False {
                    }
                    frame True {
                      n42 = call "Get Full Decay Fit & Residual Plots (1-Exp Fit).vi"("Laser Period"=w275, "Fit Options"=w276, "Error In"=w280, "Best Fit Parameters (All)"=w274, "IRF"=w282, "Full Decay"=w281) -> ("Error Out"=w279:errorcluster, "Full Decay Residuals"=w277:cluster{"t Array":dbl[], "Y Array":dbl[]}, "Full Fitted Decay"=w278:cluster{"t Array":dbl[], "Y Array":dbl[]})  [unwired: 3 in]
                    }
                  }
                }
                frame "2-Exponentials" {
                  n43 = call "AlliGator Convert New to Legacy Fit Parameter Constraints.vi"("All Parameter Constraints"=w291) -> ("Parameter Bounds"=w283:T24)
                  n44 = call "AlliGator 2-Exp + IRF Convolution Fit v2.vi"("Decay"=w294, "IRF"=w292, "Fit Options"=w288, "error in (no error)"=w303, "parameter bounds"=w283) -> ("Fitted Decay"=w299:cluster{"t Array":dbl[], "Fitted Array":dbl[]}, "Residuals"=w298:cluster{"t Array":dbl[], "Residual Array":dbl[]}, "Fit Output"=w287:T25, "Delta Best Fit Parameters"=w301:dbl[], "Guess Parameters Options"=w286:T29, "Guess Parameters"=w284:dbl[], "error out"=w296:errorcluster)  [unwired: 4 in]
                  n45 = Unbundle By Name(w287) -> ("best fit parameters"=w285:dbl[])
                  n46 = case shown="True" w300 {
                    tunnel: w299 -> [w306 _]
                    tunnel: w298 -> [w304 _]
                    tunnel: [w306 w311] -> w297
                    tunnel: w296 -> [w305 w315]
                    tunnel: [w305 w314] -> w295
                    tunnel: w293 -> [_ w313]
                    tunnel: w292 -> [_ w312]
                    tunnel: [w304 w310] -> w290
                    tunnel: w289 -> [_ w308]
                    tunnel: w288 -> [_ w309]
                    tunnel: w287 -> [_ _]
                    tunnel: w285 -> [_ w307]
                    frame False {
                    }
                    frame True {
                      n47 = call "Get Full Decay Fit & Residual Plots (2-Exp Fit).vi"("Laser Period"=w308, "Fit Options"=w309, "Error In"=w315, "Best Fit Parameters"=w307, "IRF"=w312, "Full Decay"=w313) -> ("Error Out"=w314:errorcluster, "Full Decay Residuals"=w310:cluster{"t Array":dbl[], "IRF Array":dbl[]}, "Full Fitted Decay"=w311:cluster{"t Array":dbl[], "IRF Array":dbl[]})  [unwired: 3 in]
                    }
                  }
                }
              }
            }
            frame False {
              # "New approach"
              n48 = Bundle By Name(cluster=T21 {"MLE Baseline Offset"=0.0, "MLE Baseline Offset Type"=enum."Absolute"}, "MLE Baseline Offset"=w321, "MLE Baseline Offset Type"=w320) -> (w318:T21)
              n49 = case shown="\"1-Exponential\", Default" w324 {
                tunnel: ["1-Exp Fit of " ("string") "2-Exp Fit of " ("string")] -> w333
                tunnel: [w343 w345] -> w325
                frame "1-Exponential", Default {
                  n50 = vi-ref "Fits.lvlib:LM model function and gradient (1-Exp, Convolved, Periodic, Fixed Parameters) v3.vi"() -> (w343:refnum<vi>)
                }
                frame "2-Exponentials" {
                  n51 = vi-ref "Fits.lvlib:LM model function and gradient (2-Exp, Convolved, Periodic, Fixed Parameters) v3.vi"() -> (w345:refnum<vi>)
                }
              }
              n52 = call "AlliGator n-Exp + IRF Fit v4.vi"("Decay"=w335, "VI Refnum"=w325, "IRF"=w341, "Fit Options"=w334, "MLE Fit Options"=w318, "error in (no error)"=w339, "All Parameter Constraints"=w338) -> ("All unscaled Fit Parameters (w tau)"=w316:dbl[], "Fitted Decay"=w328:cluster{"t Array":dbl[], "Fitted Array":dbl[]}, "Residuals"=w326:cluster{"t Array":dbl[], "Residual Array":dbl[]}, "Fit Output"=w317:T25, "Delta Best Fit Parameters (w tau)"=w329:dbl[], "Guess Parameters Options"=w331:T29, "Guess Parameters"=w330:dbl[], "error out"=w327:errorcluster)  [unwired: 1 in]
              n53 = case shown="True" w332 {
                tunnel: w328 -> [w349 _]
                tunnel: [w349 w356] -> w342
                tunnel: w341 -> [_ w359]
                tunnel: w340 -> [_ w358]
                tunnel: w327 -> [w348 w352]
                tunnel: [w348 w357] -> w337
                tunnel: [w347 w355] -> w336
                tunnel: w326 -> [w347 _]
                tunnel: w334 -> [_ w354]
                tunnel: w316 -> [_ w351]
                tunnel: w324 -> [_ w353]
                tunnel: w322 -> [_ w350]
                frame False {
                  # "Use data points used for fit"
                }
                frame True {
                  # "compute over full decay range"
                  n54 = case shown="\"2-Exponentials\"" w353 {
                    tunnel: w359 -> [w369 w379]
                    tunnel: w358 -> [w368 w378]
                    tunnel: [w367 w377] -> w357
                    tunnel: [w366 w376] -> w356
                    tunnel: [w365 w375] -> w355
                    tunnel: w354 -> [w364 w374]
                    tunnel: w350 -> [w363 w371]
                    tunnel: w351 -> [w362 w373]
                    tunnel: w352 -> [w361 w372]
                    frame "1-Exponential", Default {
                      n55 = call "Get Full Decay Fit & Residual Plots (1-Exp Fit) v2.vi"("SYNC Period"=w363, "Fit Options"=w364, "Use Normalized IRF (T)"=TRUE, "Error In"=w361, "Best Fit Parameters (w tau)"=w362, "IRF"=w369, "Full Decay"=w368) -> ("Error Out"=w367:errorcluster, "Full Decay Residuals"=w365:cluster{"t Array":dbl[], "Y Array":dbl[]}, "Full Fitted Decay"=w366:cluster{"t Array":dbl[], "Y Array":dbl[]})  [unwired: 2 in]
                    }
                    frame "2-Exponentials" {
                      n56 = call "Get Full Decay Fit & Residual Plots (2-Exp Fit) v2.vi"("SYNC Period"=w371, "Fit Options"=w374, "Use Normalized IRF (T)"=TRUE, "Error In"=w372, "Best Fit Parameters (w tau)"=w373, "IRF"=w379, "Full Decay"=w378) -> ("Error Out"=w377:errorcluster, "Full Decay Residuals"=w375:cluster{"t Array":dbl[], "IRF Array":dbl[]}, "Full Fitted Decay"=w376:cluster{"t Array":dbl[], "IRF Array":dbl[]})  [unwired: 2 in]
                    }
                  }
                }
              }
            }
          }
          n57 = Unbundle By Name(w158) -> ("Show Fit Residuals"=w154:bool)
          n58 = global write "Abort Fit Global.vi" "Abort Fit"(w155) -> ()
          n59 = Concatenate Strings(w157, w156) -> (w153:string)
          n60 = call "High Resolution Timing.vi"("relative seconds (NaN)"=w175, "Error In"=w180) -> ("elapsed (relative) seconds"=w170:dbl, "Error Out"=w168:errorcluster)  [unwired: 15 in, 1 out]
          n61 = case shown="True" w154 {
            tunnel: w152 -> [w222 w231]
            tunnel: [w221 w230] -> w149
            tunnel: w151 -> [_ w229]
            tunnel: w153 -> [w224 w227]
            tunnel: [w223 w225] -> w150
            frame False {
              n62 = Build Array(w224) -> (w223:string[])
              n63 = Build Array(w222) -> (w221:cluster{"t Array":dbl[], "IRF Array":dbl[]}[])
            }
            frame True {
              n64 = Build Array(w231, w229) -> (w230:cluster{"t Array":dbl[], "IRF Array":dbl[]}[])
              n65 = Concatenate Strings(w227, " Residuals" ("string")) -> (w226:string)
              n66 = Build Array(w227, w226) -> (w225:string[])
            }
          }
          n67 = case shown="True" w166 {
            tunnel: w189 -> [_ w220]
            tunnel: [w190 w206] -> w188
            tunnel: w183 -> [_ w198]
            tunnel: w173 -> [_ w216]
            tunnel: w172 -> [_ w215]
            tunnel: w156 -> [_ w203]
            tunnel: w171 -> [_ w214]
            tunnel: w159 -> [_ w213]
            tunnel: w158 -> [_ w199]
            tunnel: w164 -> [_ w212]
            tunnel: w170 -> [_ w211]
            tunnel: [_ w205] -> w169
            tunnel: w168 -> [w190 w204]
            tunnel: w165 -> [_ w202]
            tunnel: w161 -> [_ w201]
            tunnel: w160 -> [_ w200]
            tunnel: w149 -> [_ w197]
            tunnel: w150 -> [_ w196]
            tunnel: w146 -> [_ w194]
            frame False {
              # "Non-interactive Fit: Fit is not plotted"
            }
            frame True {
              # "interactive fit: Fit is plotted"
              n68 = call "AlliGator Decay Fit Output String.vi"("Plot Name"=w203, "(Clipped) Plot Range"=w216, "Plot clipped?"=w215, "All Fit Parameters"=w200, "Guess Parameters Options"=w202, "Fit Output"=w214, "Delta Best Fit Parameters"=w213, "Fit Options"=w199, "Error In"=w204, "Guess Parameters"=w201, "Fit Parameter Constraints"=w212, "CPU (s)"=w211) -> ("Fit Output Message"=w209:string, "Error Out"=w217:errorcluster)  [unwired: 2 in]
              n69 = call-poly "XY Graph Add Plot(s) with Name(s).vi"("XYGraph in"=w220, "Array of Plots"=w197, "Array of Plot Names (\"Plot\")"=w196, "error in (no error)"=w217, "Plot Colors (Default)"=w198) -> ("XY Graph Caption"=w192:string, "Added Plot Names"=w219:string[], "error out"=w207:errorcluster)  [unwired: 6 in, 2 out]
              n70 = call "Concatenate String Array.vi"("Separator (TAB)"=", ", "String Array"=w219) -> ("Formatted String"=w208:string)  [unwired: 9 in]
              n71 = Select(t="\nLegacy Approach\n", s=w194, f="") -> (s? t:f=w191:string)
              n72 = Format Into String(format string="%s\nPlot(s) added to %s: %s", initial string=w209, error in=w207, w191, w192, w208) -> (resulting string=w205:string, error out=w206:errorcluster)
            }
          }
          n73 = Unbundle By Name(w171) -> ("covariance"=w177:T17)
          n74 = Unbundle By Name(w171) -> ("R^2"=w179:dbl, "Chi 2"=w178:dbl, "DOF"=w162:i32)
          n75 = Compound Arithmetic op=MULTIPLY(w178, invert w162) -> (w163:dbl)
        }
        frame Error {
          w381 = nan ("element")
          # "If decay is not valid, no plot is added to the Graph and NaN parameters are returned"
          n76 = case shown="\"1-Exponential\", Default" w384 {
            tunnel: [4 ("dimension size") 6 ("dimension size")] -> w383
            frame "1-Exponential", Default {
            }
            frame "2-Exponentials" {
            }
          }
          n77 = Initialize Array(w381, w383) -> (w382:dbl[])
        }
      }
    }
  }
  "Error Out" <- w35
  "Fit Output Message" <- w34
  "Best Fit Parameters (All)" <- w33
  "Delta Best Fit Parameters (All)" <- w32
  "R^2" <- w31
  "Reduced Chi^2" <- w30
  "Covariance" <- w22
  "Decay Fit Options & Parameters (out)" <- w8
  "Output Plots" <- w2
  "Output Plot Names" <- w1
